vi "Pulse DC Voltage.vi"(8 "error in (no error)":errorcluster, 10 "Params":variant, 11 "NI SMU in":refnum<class "NI SMU.lvclass">) -> (0 "error out":errorcluster, 3 "NI SMU out":refnum<class "NI SMU.lvclass">)   [LabVIEW 2020, in "NI SMU.lvlib" / "NI SMU.lvclass"]
uses:
  NI SMU.lvclass
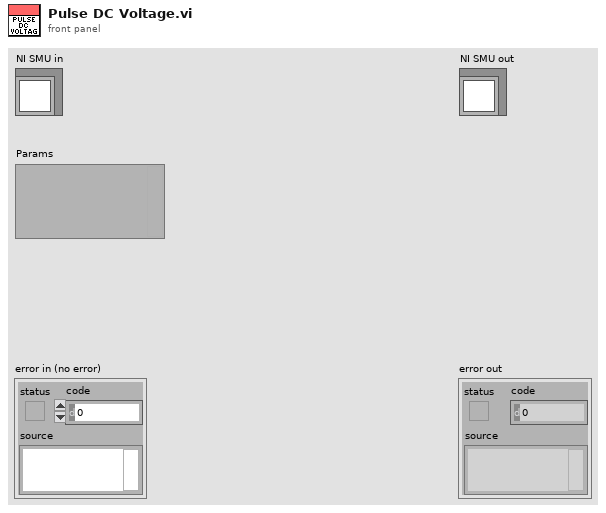
[diagram p1: front panel]
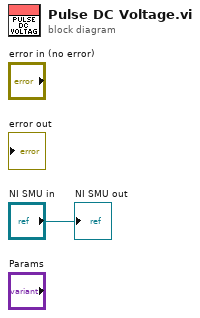
[diagram p0: block diagram]
diagram:
  "NI SMU out" <- "NI SMU in"
